vi "set Color.vi"(8 "error in (no error)":errorcluster, 9 "Color style":T1, 10 "style index":i32, 11 "ScintillaNET in":refnum<class "ScintillaNET.lvclass">) -> (0 "error out":errorcluster, 3 "ScintillaNET out":refnum<class "ScintillaNET.lvclass">)   [LabVIEW 2018, in "ScintillaNET.lvclass"]
uses:
  ScintillaNET.lvclass
  ScintillaNET.lvclass/ScintillaNET.ctl
  D:/project/hobby/LF2R/LabVIEW/source/ScintillaNET/dll/ScintillaNET.dll
  dll/ScintillaNET.dll
  System.Drawing
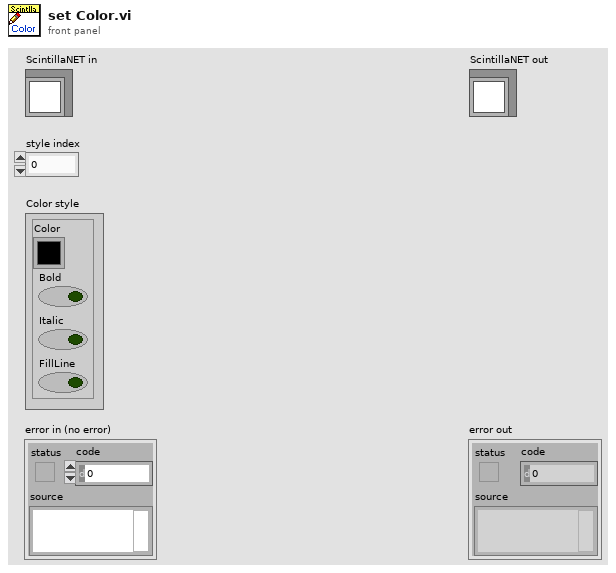
[diagram p1: front panel]
types:
  T1 = cluster{"Color":u32, "Bold":bool, "Italic":bool, "FillLine":bool}
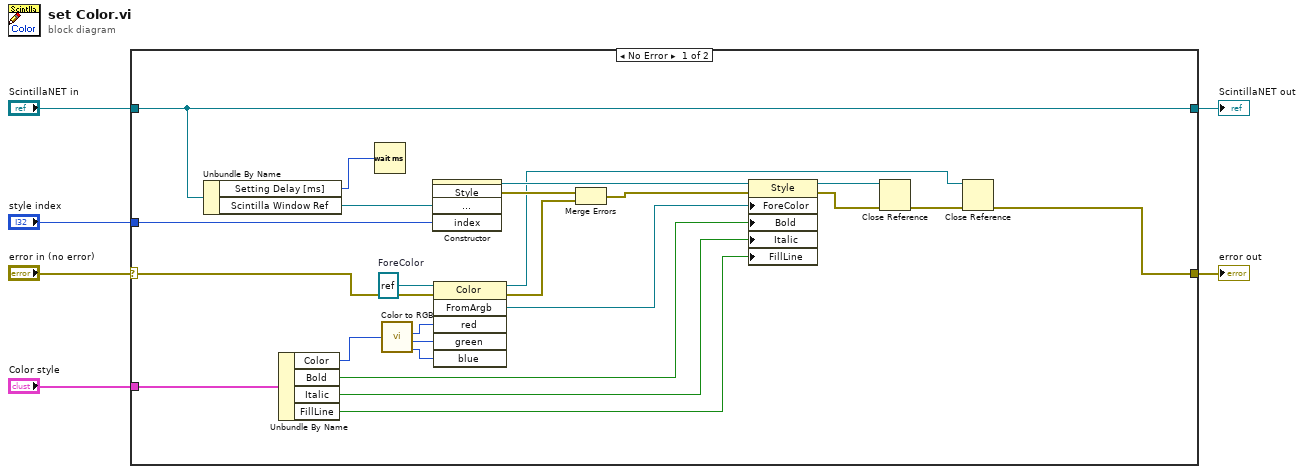
[diagram p0: block diagram]
diagram:
  n1 = case shown="No Error" "error in (no error)" {
    selector: "error in (no error)" -> [w8 w32]
    tunnel: [w10 w32] -> w5
    tunnel: [w21 w31] -> w3
    tunnel: "ScintillaNET in" -> [w21 w31]
    tunnel: "Color style" -> [w17 _]
    tunnel: "style index" -> [w9 _]
    frame No Error {
      w29 = refnum<k24> refnum  # ForeColor
      n2 = Unbundle By Name(w21) -> ("Setting Delay [ms]"=w7:u32, "Scintilla Window Ref"=w22:refnum<k24>)
      n3 = Unbundle By Name(w17) -> ("Color"=w16:u32, "Bold"=w20:bool, "Italic"=w19:bool, "FillLine"=w18:bool)
      n4 = Wait (ms)(milliseconds to wait=w7) -> ()  [unwired: 1 out]
      n5 = call <vilib>:"Color to RGB.vi"("Color"=w16) -> ("R"=w28:u8, "G"=w27:u8, "B"=w26:u8)  [unwired: 1 out]
      n6 = constructor class="Style"("scintilla"=w22, "index"=w9) -> (reference out=w30:refnum<k24>, error out=w14:errorcluster)  [unwired: 3 in, 3 out]
      n7 = invoke class="Color" method="FromArgb"(reference=w29, error in=w8, "red"=w28, "green"=w27, "blue"=w26) -> (reference out=w11:refnum<k24>, error out=w15:errorcluster, "FromArgb"=w25:refnum<k24>)  [unwired: 1 in, 3 out]
      n8 = Merge Errors(w14, w15) -> (w13:errorcluster)
      n9 = property class="Style"(reference=w30, error in=w13, "ForeColor"=w25, "Bold"=w20, "Italic"=w19, "FillLine"=w18) -> (reference out=w24:refnum<k24>, error out=w23:errorcluster)
      n10 = Close Reference(reference=w24, error in (no error)=w23) -> (error out=w12:errorcluster)
      n11 = Close Reference(reference=w11, error in (no error)=w12) -> (error out=w10:errorcluster)
    }
    frame Error {
    }
  }
  "error out" <- w5
  "ScintillaNET out" <- w3
